vi "QMH Check Queue Status.vi"(7 "error in (no error)":errorcluster, 10 "queue in":refnum<queue>) -> (0 "error out":errorcluster, 2 "# elements in queue":i32, 3 "queue out":refnum<queue>)   [LabVIEW 2013, in "QHM.lvlib"]
uses:
  QHM.lvlib
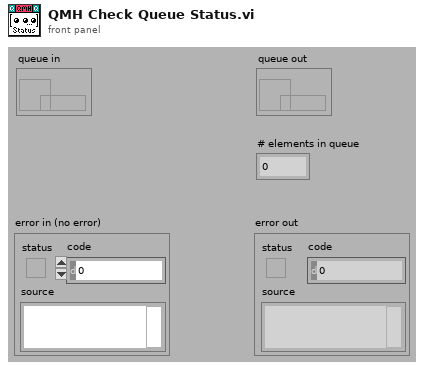
[diagram p1: front panel]
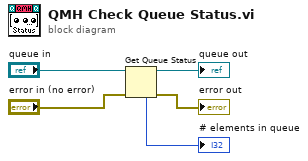
[diagram p0: block diagram]
diagram:
  n1 = Get Queue Status(queue="queue in", error in (no error)="error in (no error)") -> (queue out=→"queue out":refnum<queue>, error out=→"error out":errorcluster, # elements in queue=→"# elements in queue":i32)  [unwired: 1 in, 5 out]
